vi "Constructor.vi"(8 "error in":errorcluster, 11 "Detector in":refnum<class "PID.lvclass">) -> (0 "error out":errorcluster, 2 "init":bool, 3 "Detector out":refnum<class "PID.lvclass">)   [LabVIEW 2011, in "PID.lvclass"]
doc: "Initialisation of the spectral detector and allocation of software recourses to variables registered by Detector.ctl."
uses:
  PID.lvclass
  PID.lvclass/PID.ctl
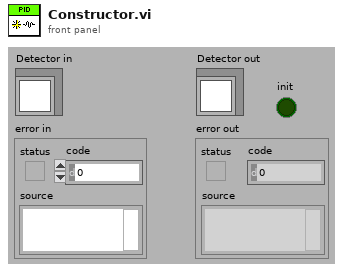
[diagram p1: front panel]
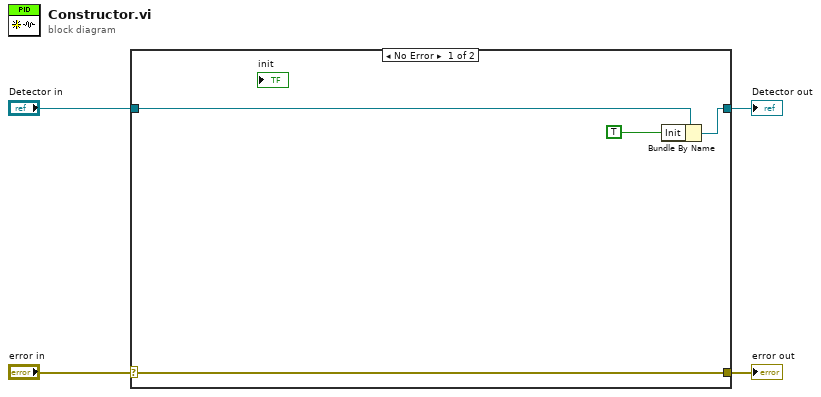
[diagram p0: block diagram]
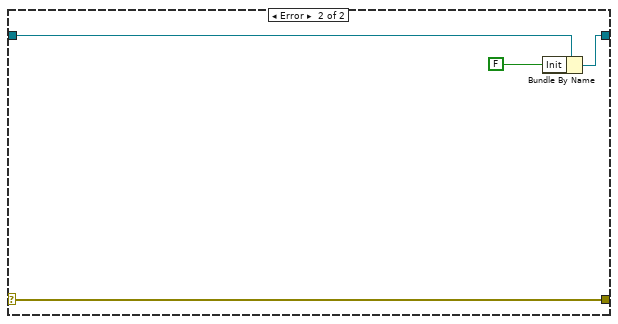
[diagram p2: hidden frame]
diagram:
  n1 = case shown="No Error" "error in" {
    selector: "error in" -> [w8 w12]
    tunnel: [w8 w12] -> w3
    tunnel: [w6 w9] -> w1
    tunnel: "Detector in" -> [w7 w11]
    frame No Error {
      n2 = Bundle By Name(cluster=w7, "Init"=TRUE) -> (w6:refnum<class "PID.lvclass">)
    }
    frame Error {
      n3 = Bundle By Name(cluster=w11, "Init"=FALSE) -> (w9:refnum<class "PID.lvclass">)
    }
  }
  "error out" <- w3
  "Detector out" <- w1
